vi "replaces_instances.vi"(8 "error in (no error)":errorcluster, 9 "instances":refnum<data-value>[](array[refnum]), 10 "Base Class (LabVIEW Object)":refnum<class>, 11 "Default Lookup in":refnum<class "Default Lookup.lvclass">) -> (0 "error out":errorcluster, 3 "Default Lookup out":refnum<class "Default Lookup.lvclass">)   [LabVIEW 2014, in "LVCOOOP.lvlib" / "Lookup API.lvlib" / "Default Lookup.lvclass"]
uses:
  Default Lookup.lvclass
  Default Lookup.lvclass/Default Lookup.ctl
  types/lookup_data.ctl
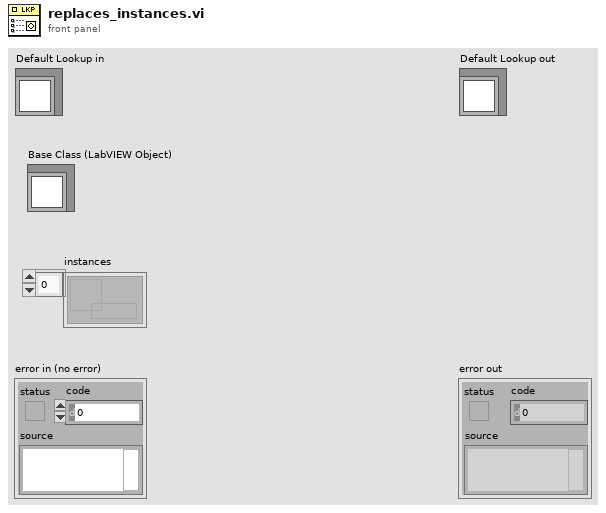
[diagram p1: front panel]
types:
  T1 = typedef "LVCOOOP.lvlib/Lookup API.lvlib/Default Lookup.lvclass/lookup_data.ctl" = cluster{"instances":refnum<data-value>[], "listeners":refnum<user-event>[]}
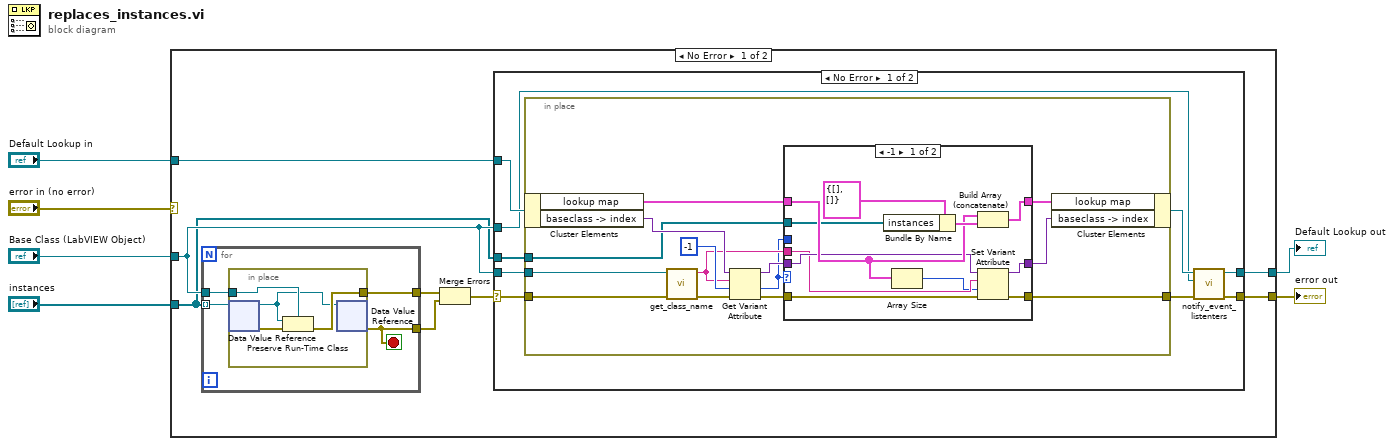
[diagram p0: block diagram]
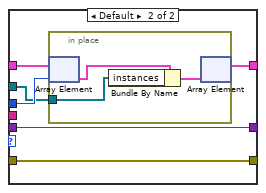
[diagram p2: hidden frame]
diagram:
  n1 = case shown="No Error" "error in (no error)" {
    selector: "error in (no error)" -> [_ w69]
    tunnel: [w9 w69] -> w2
    tunnel: "instances" -> [w7 _]
    tunnel: "Base Class (LabVIEW Object)" -> [w8 _]
    tunnel: "Default Lookup in" -> [w11 w68]
    tunnel: [w10 w68] -> w1
    frame No Error {
      n2 = for {
        tunnel: w7 -> [w18] mode=indexing
        tunnel: [w17] -> w14
        tunnel: [w15] -> w13
        tunnel: w8 -> [w16]
        stop <- w15 stop-if-true
        n3 = in-place {
          in-place-border: w16 -> [w22]
          in-place-border: [w20] -> w17
          n4 = in-place-dvr #1(w18) -> (w19:refnum<class>, w21:errorcluster)
          n5 = Preserve Run-Time Class(object in=w19, error in=w21, 2:w22) -> (error out=w20:errorcluster)  [unwired: 1 out]
          n6 = in-place-dvr #1(w19) -> (w15:errorcluster)  [unwired: 1 out]
        }
      }
      n7 = Merge Errors(w14, w13) -> (w12:errorcluster)
      n8 = case shown="No Error" w12 {
        selector: w12 -> [w29 w66]
        tunnel: w11 -> [w31 w67]
        tunnel: w8 -> [w30 _]
        tunnel: w7 -> [w28 _]
        tunnel: [w24 w67] -> w10
        tunnel: [w25 w66] -> w9
        tunnel: w8 -> [w23 _]
        frame No Error {
          n9 = in-place {
            in-place-border: w30 -> [w44]
            in-place-border: w29 -> [w43]
            in-place-border: w28 -> [w39]
            in-place-border: [w32] -> w26
            n10 = in-place-cluster #2(w31) -> ("lookup map"=w40:T1[], "baseclass -> index"=w45:variant)
            n11 = call "get_class_name.vi"("error in (no error)"=w43, "LabVIEW Object in"=w44) -> ("error out"=w42:errorcluster, "class name"=w36:string)  [unwired: 8 in]
            n12 = Get Variant Attribute(Variant=w45, name=w36, default value (empty Variant)=-1, error in=w42) -> (duplicate Variant=w37:variant, value=w33:i32, error out=w35:errorcluster)  [unwired: 1 out]
            n13 = case shown="-1" w33 {
              tunnel: w40 -> [w53 w62]
              tunnel: w39 -> [w46 w59]
              tunnel: [w54 w61] -> w38
              tunnel: w37 -> [w52 w58]
              tunnel: w36 -> [w51 _]
              tunnel: w35 -> [w49 w57]
              tunnel: [w48 w58] -> w34
              tunnel: w33 -> [_ w60]
              tunnel: [w47 w57] -> w32
              frame -1 {
                n14 = Bundle By Name(cluster=T1 {"instances"=[], "listeners"=[]} ("lookup data"), "instances"=w46) -> (w55:T1)
                n15 = Array Size(array=w53) -> (size(s)=w50:i32)
                n16 = Build Array (concatenate)(w53, w55) -> (w54:T1[])
                n17 = Set Variant Attribute(Variant=w52, name=w51, value=w50, error in=w49) -> (Variant out=w48:variant, error out=w47:errorcluster)  [unwired: 1 out]
              }
              frame Default {
                n18 = in-place {
                  in-place-border: w59 -> [w64]
                  n19 = in-place-array #3(w62, w60) -> (w65:T1)
                  n20 = Bundle By Name(cluster=w65, "instances"=w64) -> (w63:T1)
                  n21 = in-place-array #3(w63) -> (w61:T1[])  [unwired: 1 out]
                }
              }
            }
            n22 = in-place-cluster #2("lookup map"=w38, "baseclass -> index"=w34) -> (w27:refnum<class "Default Lookup.lvclass">)
          }
          n23 = call-dynamic "notify_event_listenters.vi"("error in (no error)"=w26, "Base Class (LabVIEW Object)"=w23, "Default Lookup in"=w27) -> ("error out"=w25:errorcluster, "Default Lookup out"=w24:refnum<class "Default Lookup.lvclass">)  [unwired: 7 in]
        }
        frame Error {
        }
      }
    }
    frame Error {
    }
  }
  "error out" <- w2
  "Default Lookup out" <- w1
